vi "SEA_9811_Close.vi"(8 "error in (no error)":errorcluster, 11 "SEA9811_RT_data in":T1) -> (0 "error out":errorcluster)   [LabVIEW 2012]
uses:
  Typdefs/SEA9811_RT_data_cluster.ctl
  <userlib>/_FPGA Interface Advanced Tools/FPGA Interface Base/FPGA Interface Base.lvclass
  Typdefs/FPGA ref.ctl
  Typdefs/channel.ctl
  Typdefs/received word.ctl
  Typdefs/SEA9811_FPGA_FP_Addresses.ctl
  <userlib>/_FPGA Interface Advanced Tools/FPGA Interface Wrapper/TypeDefs/Close Attribute.ctl
  <userlib>/_FPGA Interface Advanced Tools/FPGA Interface Wrapper/FPGA Interface Wrapper.lvlib
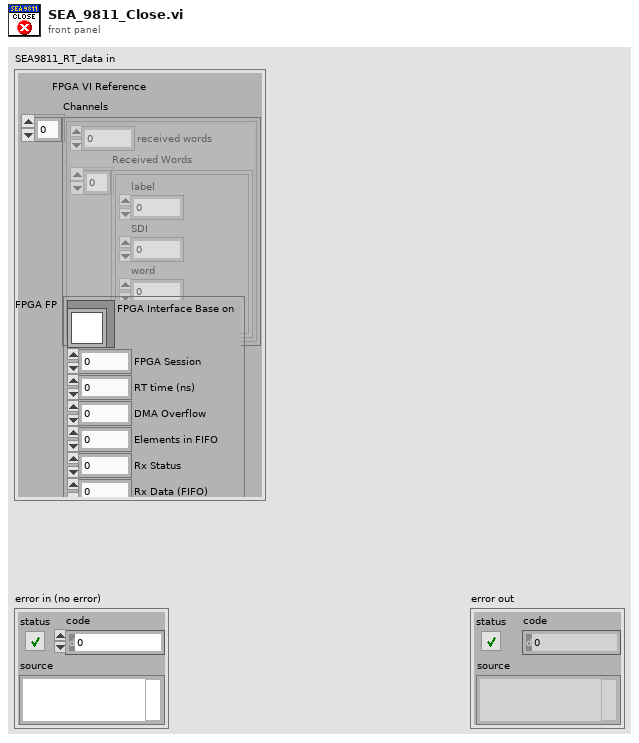
[diagram p1: front panel]
types:
  T1 = typedef "SEA9811_RT_data_cluster.ctl" = cluster{"FPGA VI Reference":T2, "Channels":T3[], "FPGA FP":T5}
  T2 = typedef "FPGA ref.ctl" = refnum<k20>
  T3 = typedef "channel.ctl" = cluster{"received words":u32, "Received Words":T4[]}
  T4 = typedef "received word.ctl" = cluster{"label":u8, "SDI":u8, "word":u32, "timestamp":dbl}
  T5 = typedef "SEA9811_FPGA_FP_Addresses.ctl" = cluster{"FPGA Interface Base on":refnum<class "FPGA Interface Base.lvclass">, "FPGA Session":u32, "RT time (ns)":u32, "DMA Overflow":u32, "Elements in FIFO":u32, "Rx Status":u32, "Rx Data (FIFO)":u32}
  T6 = typedef "FPGA Interface Wrapper.lvlib/Close Attribute.ctl" = enum32{"Reset if Last Session (Default)", "No Reset"}
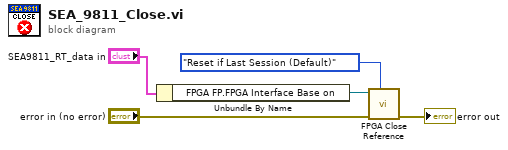
[diagram p0: block diagram]
diagram:
  n1 = Unbundle By Name("SEA9811_RT_data in") -> ("FPGA FP.FPGA Interface Base on"=w2:refnum<class "FPGA Interface Base.lvclass">)
  n2 = call-dynamic "FPGA Close Reference.vi"("Reset?"=Close_Attribute."Reset if Last Session (Default)", "error in (no error)"="error in (no error)", "FPGA Session In"=w2) -> ("error out"=→"error out":errorcluster)  [unwired: 8 in]
